vi "Initialize.vi"(8 "error in (no error)":errorcluster, 10 "Baud Rate (115200)":u32=115200, 11 "VISA resource name":refnum<visa-resource-name>) -> (0 "error out":errorcluster, 3 "VISA resource name out":refnum<visa-resource-name>)   [LabVIEW 2013, in "Zaber A Series.lvlib"]
doc: "Establishes communication with a Zaber device and clears teh serial buffer. Call this VI before calling other instrument driver VIs for this instrument. You need to call the Initialize VI only once at the beginning of an application, or again after using the Close VI. \n\nNote: \nThe default baud rate for the ASCII protocol is 115200, but the devices can be adjusted to use different baud rates in which case you should adjust the baud rate indicator."
uses:
  Zaber A Series.lvlib
  <vilib>/Instr/_visa.llb/VISA Configure Serial Port (Instr).vi
panel:
  # "(c) 2014 Zaber Technologies.  ALL RIGHTS RESERVED."
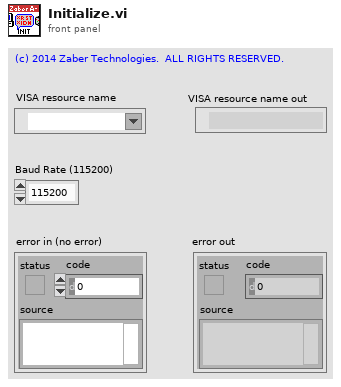
[diagram p1: front panel]
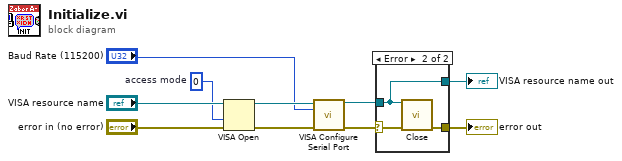
[diagram p0: block diagram]
diagram:
  w8 = u32 0  # access mode
  n1 = VISA Open(access mode=w8, error in (no error)="error in (no error)", VISA resource name="VISA resource name") -> (VISA resource name=w2:refnum<visa-resource-name>, error out=w3:errorcluster)  [unwired: 2 in]
  n2 = call-poly "VISA Configure Serial Port"("VISA resource name"=w2, "baud rate (9600)"="Baud Rate (115200)", "error in (no error)"=w3) -> ("VISA resource name out"=w5:refnum<visa-resource-name>, "error out"=w4:errorcluster)  [unwired: 11 in]
  n3 = case shown="Error" w4 {
    selector: w4 -> [w11 w14]
    tunnel: w5 -> [w12 w13]
    tunnel: [w12 w13] -> w7
    tunnel: [w11 w15] -> w6
    frame No Error {
    }
    frame Error {
      n4 = call "Close.vi"("error in (no error)"=w14, "VISA resource name"=w13) -> ("error out"=w15:errorcluster)  [unwired: 9 in]
    }
  }
  "VISA resource name out" <- w7
  "error out" <- w6
